vi "moveOne.vi"(6 "Which mono":enum16{"Mono 1", "Mono 2"}(ring), 7 "Monochromator":T1={"Type"=enum."PTI", "Wavelength (nm)"=600.0, "Grating, gr/mm"=enum."1200", "Grating mode"=enum."Unknown", "Spectrum mode"={"Spectrum mode?"=FALSE, "Start wavelength (nm)"=0.0, "End wavelength (nm)"=0.0, "Wavelength step (nm)"=0.0, "Wavelength array"=[], "array index"=0}, "PTI"={"Delay before read (ms)"=50, "Mono 1"={"Timeout (ms)"=1000, "Resource Name"="COM1", "Baud Rate"=9600, "Data Bits"=8, "Parity"=0, "Stop Bits"=10, "Flow Control"=0}, "Mono 2"={"Timeout (ms)"=1000, "Resource Name"="COM1", "Baud Rate"=9600, "Data Bits"=8, "Parity"=0, "Stop Bits"=10, "Flow Control"=0}, "Two PTI Monochromators?"=FALSE}, "Oriel (custom)"={"reference"=refnum}, "Force wavelength confirmation (PTI)?"=FALSE} {"PTI"."Mono 2"."Flow Control" items=["1.0"=10, "1.5"=15, "2.0"=20]; "PTI"."Mono 2"."Stop Bits" items=["None", "Odd", "Even", "Mark", "Space"]; "PTI"."Mono 2"."Parity" items=["None", "Odd", "Even", "Mark", "Space"]; "PTI"."Mono 1"."Flow Control" items=["1.0"=10, "1.5"=15, "2.0"=20]; "PTI"."Mono 1"."Stop Bits" items=["None", "Odd", "Even", "Mark", "Space"]; "PTI"."Mono 1"."Parity" items=["None", "Odd", "Even", "Mark", "Space"]}, 8 "error in (no error)":errorcluster={"status"=FALSE, "code"=-1073807346, "source"=""}, 10 "Debug messages?":bool, 11 "Delta wavelength (nm)":dbl=-100.0 format="%.3f") -> (0 "error out":errorcluster={"status"=TRUE, "code"=-1073807343, "source"="VISA Write in Monochromator.lvlib:move.vi"})   [LabVIEW 2017, in "Monochromator.lvlib" / "PTI.lvlib"]
doc: "The Advanced Serial Read and Write example performs a Serial Port Read, a Serial Port Write, or a combination of these actions while setting some advanced serial features like buffer size, termination characters, and XON/XOFF flow control. The user selects the actions (read or write) on the front panel. If both are selected, the VI will write the data first, read the data and then close the VISA session that is opened to the port. \n\nThe parameters set for the serial port must match the parameters of the connected instrument or device. In this example, the bytes to read parameter specifies the number of bytes that the serial port reads. If there were more bytes at the port than the number specified in bytes to read, those bytes would not be read. Also, if you specify to read more bytes than the number of bytes actually read, you might receive a timeout error message.\n\nINSTRUCTIONS:\n1) Select the serial resource and configuration parameters (baud rate, data bits, parity, stop bits, flow control).\n2) Termination character can be enabled and set. Also, set the required input buffer size prior to running the example.\n3) Select the operations to be performed. \n4) Connect the serial port to your device. If no device is available, perform a loopback test by doing one of the following. Short pins 2 and 3 on a RS-232 cable or short pin 4 to pin 8 and pin 5 to pin 9 on a RS-485/422 cable. \n5) Run the VI to see the data read. (The \"read string\" will match the \"string to write\" if a loopback test was performed.)\n\nThis example exposes several advanced features that you may need for your application. Not all applications need all the features shown in this example. The input buffer size is likely an important setting that you want to control in your application. This example expands upon the flow control option for XON and XOFF, allowing the user to choose those control characters. The timeout parameter has been brought to the front panel so a user can specify the time period the VISA Read will wait for the number of bytes to read before timing out. Also, the user has several controls for the termination character, which is discussed later.\n\nNote that you can press the write and read buttons and change the bytes to read parameters on the fly, while the example is running. However, you must stop the example to change the other configuration parameters after the example has started running, and then run again.\n\nSet the I/O buffer size slightly higher the amount of data you expect to receive. This is very important for applications that don't use flow control, as you may lose characters if the receive buffer overflows.\n\nSetting the timeout period ensures that the operation returns with a timeout error if the operation cannot be performed in the specified time period. \n\nSome devices require a termination character in order to identify the end of command strings. Some devices send a termination character to signify the end of data to be read. \n\nThis example shows how you can end the Read operation once a termination character is detected in the buffer and/or append a termination character at the end of the Write data. To enable the Read to end on a termination character, use the VISA Configure Serial Port or use the VISA Properties Serial End Mode for Reads, Termination Character Enable, and Termination Character. To end the Write with a termination character, use the VISA Properties Serial End Mode for Writes, the Send End Enable, and Termination Character. In this example, the same termination character is used for both the Read and the Write. You can specify two different characters for your application, if desired.\n\nYour application may require specific characters for the XON/XOFF Flow Control. You can specify these characters with the VISA Properties Flow Control XOFF Character and Flow Control XON Character. Note that if the standard XON and XOFF characters are used, then decimal 17 and 19 are unavailable for data values. Remember that using flow control and setting an adequate buffer size allow you to prevent buffer overflows."
uses:
  PTI.lvlib
  Controls/Params.ctl
  Controls/Type.ctl
  Controls/GratingValues.ctl
  Controls/Grating.ctl
  Controls/VISA parameters.ctl
  Custom Oriel drivers/Controls/Params.ctl
  C:/Project Work/icl-optical-software-rewrite/Optical Software Code Simplified/Modules/Monochromator/Cornerstone.dll
  Cornerstone.dll
  Monochromator.lvlib
  Serial comms/Serial comms.lvlib
  Custom Oriel drivers/Oriel (custom drivers).lvlib
panel:
  out "Command":string
  out "move":bool=TRUE
  out "delay":bool
  out "move done":bool
  out "bytes to read":u32
  out "string 2":string
  out "Loop":i32
  in  "stop":bool
  # "nm"
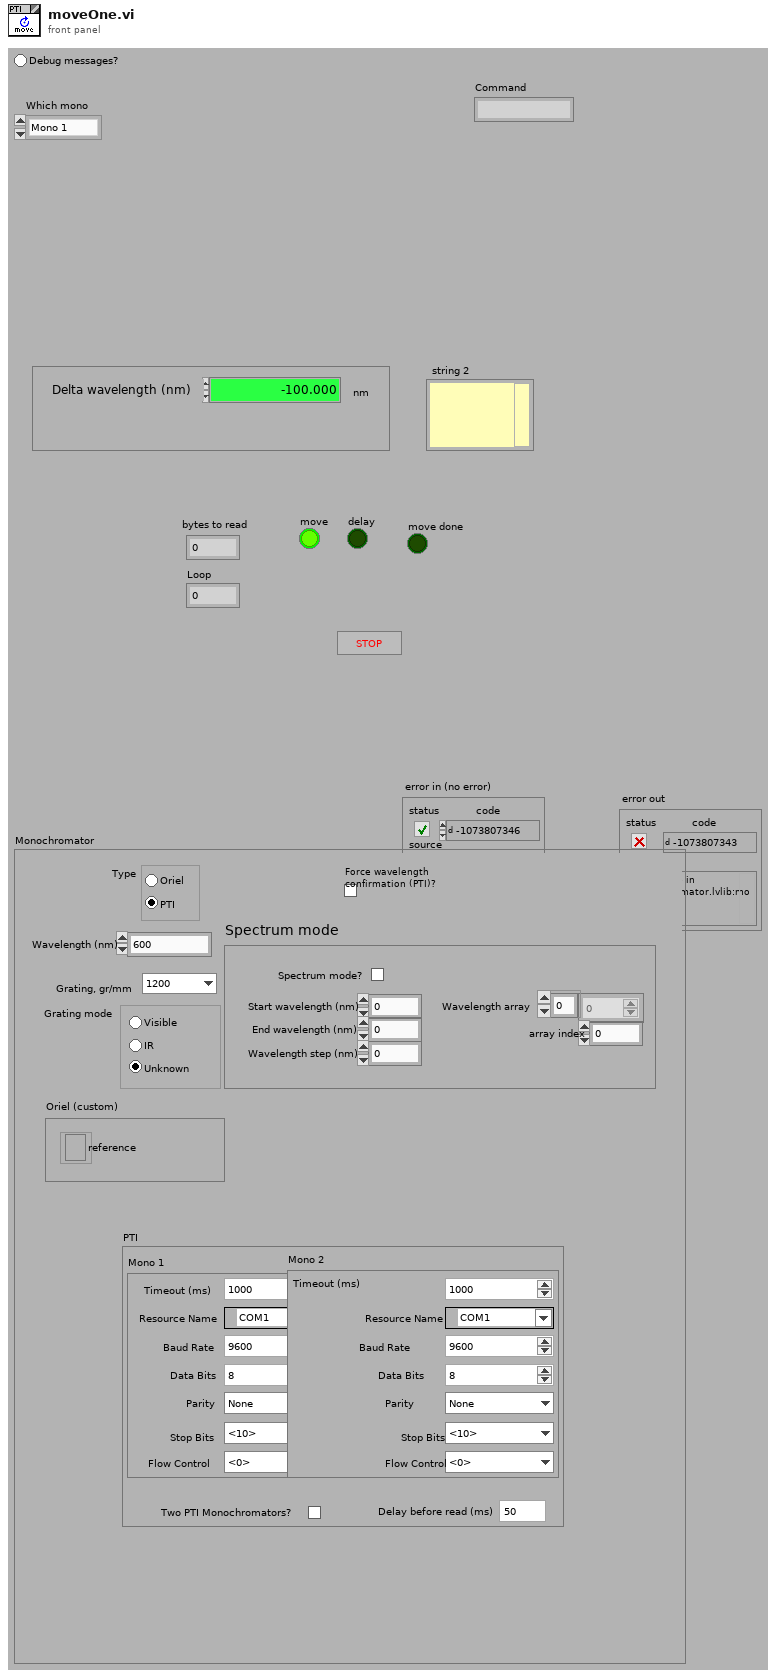
[diagram p1: front panel]
types:
  T1 = typedef "Monochromator.lvlib/Params.ctl" = cluster{"Type":T2, "Wavelength (nm)":dbl, "Grating, gr/mm":T3, "Grating mode":T4, "Spectrum mode":cluster{"Spectrum mode?":bool, "Start wavelength (nm)":dbl, "End wavelength (nm)":dbl, "Wavelength step (nm)":dbl, "Wavelength array":dbl[], "array index":u32}, "PTI":T5, "Oriel (custom)":T7, "Force wavelength confirmation (PTI)?":bool}
  T2 = typedef "Monochromator.lvlib/Type.ctl" = enum32{"Oriel", "PTI"}
  T3 = typedef "Monochromator.lvlib/GratingValues.ctl" = enum16{"2400", "1800", "1200", "600", "300", "150"}
  T4 = typedef "Monochromator.lvlib/Grating.ctl" = enum32{"Unknown", "Visible", "IR"}
  T5 = typedef "Monochromator.lvlib/PTI.lvlib/Params.ctl" = cluster{"Delay before read (ms)":u32, "Mono 1":T6, "Mono 2":T6, "Two PTI Monochromators?":bool}
  T6 = typedef "Serial comms.lvlib/VISA parameters.ctl" = cluster{"Timeout (ms)":u32, "Resource Name":refnum<visa-resource-name>, "Baud Rate":u32, "Data Bits":u16, "Parity":u16, "Stop Bits":u16, "Flow Control":u16}
  T7 = typedef "Monochromator.lvlib/Oriel (custom drivers).lvlib/Params.ctl" = cluster{"reference":refnum<k24>}
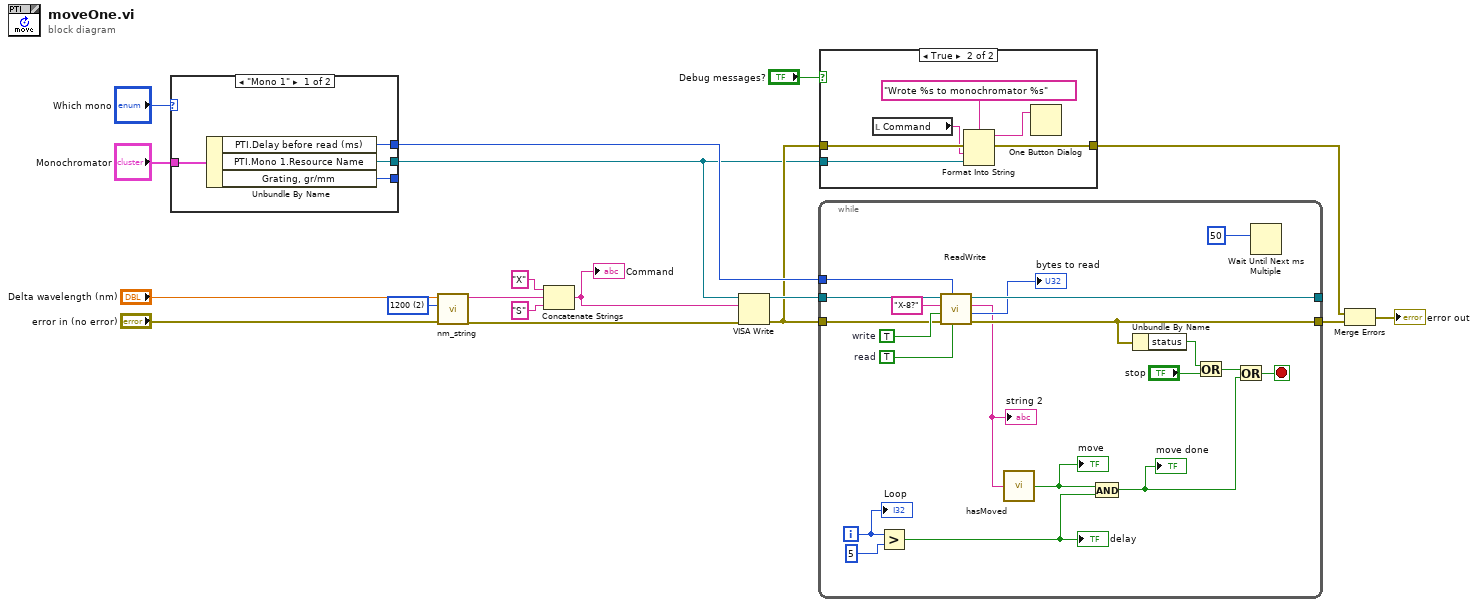
[diagram p0: block diagram]
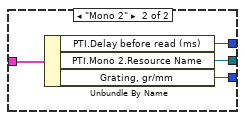
[diagram p3: hidden frame]
diagram:
  w1 = u16 2 items=["2400", "1800", "1200", "600", "300", "150"] ("Grating, gr/mm")
  n1 = case shown="\"Mono 1\"" "Which mono" {
    tunnel: "Monochromator" -> [w22 w26]
    tunnel: [w21 w25] -> w6
    tunnel: [w20 w24] -> w8
    tunnel: [w19 w23] -> _
    frame "Mono 1" {
      n2 = Unbundle By Name(w22) -> ("PTI.Delay before read (ms)"=w20:u32, "PTI.Mono 1.Resource Name"=w21:refnum<visa-resource-name>, "Grating, gr/mm"=w19:T3)
    }
    frame "Mono 2" {
      n3 = Unbundle By Name(w26) -> ("PTI.Delay before read (ms)"=w24:u32, "PTI.Mono 2.Resource Name"=w25:refnum<visa-resource-name>, "Grating, gr/mm"=w23:T3)
    }
  }
  n4 = call "nm_string.vi"("error in (no error)"="error in (no error)", "Grating, gr/mm"=w1, "Wavelength, nm"="Delta wavelength (nm)") -> ("error out"=w14:errorcluster, "nm_String"=w16:string)  [unwired: 7 in]
  n5 = Concatenate Strings("X" ("string"), w16, "S" ("string")) -> (w11:string)
  "Command" <- w11
  n6 = VISA Write(VISA resource name=w6, write buffer=w11, error in (no error)=w14) -> (VISA resource name out=w12:refnum<visa-resource-name>, error out=w7:errorcluster)  [unwired: 1 out]
  n7 = while {
    tunnel: [w46] -> _
    tunnel: [w45] -> w4
    tunnel: w12 -> [w41]
    tunnel: w7 -> [w28]
    tunnel: w8 -> [w27]
    i -> [w34]
    stop <- w39 stop-if-true
    w36 = TRUE  # read
    w37 = TRUE  # write
    n8 = Greater?(x=w34, y=5 ("x")) -> (0:w29:bool)
    "delay" <- w29
    n9 = call "ReadWrite.vi"("read"=w36, "delay before read (ms)"=w27, "error in"=w28, "write"=w37, "string to write"="X-8?", "VISA  name in"=w41) -> ("error out"=w45:errorcluster, "bytes to read"=→"bytes to read":u32, "read string"=w32:string, "VISA out"=w46:refnum<visa-resource-name>)
    "string 2" <- w32
    n10 = call "hasMoved.vi"("read string 2"=w32) -> ("move"=w30:bool)
    "move" <- w30
    n11 = And(x=w30, y=w29) -> (x .and. y?=w31:bool)
    "move done" <- w31
    n12 = Unbundle By Name(w45) -> ("status"=w44:bool)
    n13 = Or(x=w44, y="stop") -> (x .or. y?=w40:bool)
    n14 = Or(x=w40, y=w31) -> (x .or. y?=w39:bool)
    n15 = Wait Until Next ms Multiple(millisecond multiple=u32 50) -> ()  [unwired: 1 out]
    "Loop" <- w34
  }
  n16 = case shown="True" "Debug messages?" {
    tunnel: w7 -> [w47 w51]
    tunnel: [w47 w50] -> w3
    tunnel: w6 -> [_ w49]
    frame False {
    }
    frame True {
      n17 = local read "Command"() -> (w48:string)
      n18 = Format Into String(format string="Wrote %s to monochromator %s", error in=w51, w48, w49) -> (resulting string=w53:string, error out=w50:errorcluster)  [unwired: 1 in]
      n19 = One Button Dialog(message=w53) -> ()  [unwired: 1 in, 1 out]
    }
  }
  n20 = Merge Errors(w3, w4) -> (→"error out":errorcluster)
